vi "Get Attributes.vi"(8 "error in (no error)":errorcluster, 11 "Tone in":refnum<class "Tone.lvclass">) -> (0 "error out":errorcluster, 2 "Attributes":T1={"Spectrum"=FALSE, "Gate"=TRUE, "Mod"=TRUE, "Filter"=FALSE}, 3 "Tone out":refnum<class "Tone.lvclass">)   [LabVIEW 2020, in "Tone.lvclass"]
uses:
  Tone.lvclass
  Waveform/Attributes.ctl
  Waveform/Waveform.lvclass
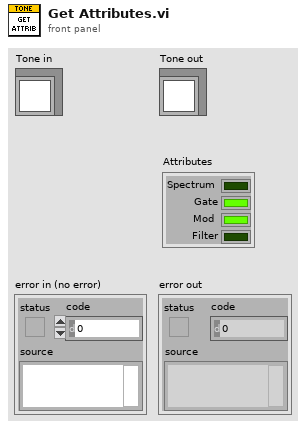
[diagram p1: front panel]
types:
  T1 = typedef "Waveform.lvclass/Attributes.ctl" = cluster{"Spectrum":bool, "Gate":bool, "Mod":bool, "Filter":bool}
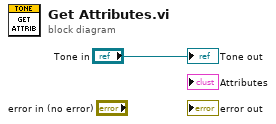
[diagram p0: block diagram]
diagram:
  "Tone out" <- "Tone in"
